vi "GetProbePlanCoordinates.vi"(8 "Use index as X coord":bool=TRUE, 9 "Probe Card Channels":i32=1) -> (0 "file path":string, 2 "OK?":bool, 3 "Array":T1(array[cluster]))   [LabVIEW 2018] (continued)
X=102970.01\ty=15800.93 \nLabel=Strip\t776\tX=103316.84\ty=15902.32 \nLabel=Strip\t777\tX=102964.55\ty=15968.32 \nLabel=Strip\t778\tX=103311.35\ty=16069.84 \nLabel=Strip\t779\tX=102959.04\ty=16135.72 \nLabel=Strip\t780\tX=103305.80\ty=16237.35 \nLabel=Strip\t781\tX=102953.46\ty=16303.11 \nLabel=Strip\t782\tX=103300.19\ty=16404.87 \nLabel=Strip\t783\tX=102947.83\ty=16470.51 \nLabel=Strip\t784\tX=103294.52\ty=16572.38 \nLabel=Strip\t785\tX=102942.14\ty=16637.90 \nLabel=Strip\t786\tX=103288.80\ty=16739.89 \nLabel=Strip\t787\tX=102936.40\ty=16805.30 \nLabel=Strip\t788\tX=103283.02\ty=16907.41 \nLabel=Strip\t789\tX=102930.59\ty=16972.69 \nLabel=Strip\t790\tX=103277.18\ty=17074.92 \nLabel=Strip\t791\tX=102924.73\ty=17140.08 \nLabel=Strip\t792\tX=103271.28\ty=17242.43 \nLabel=Strip\t793\tX=102918.81\ty=17307.47 \nLabel=Strip\t794\tX=103265.33\ty=17409.94 \nLabel=Strip\t795\tX=102912.84\ty=17474.86 \nLabel=Strip\t796\tX=103259.32\ty=17577.45 \nLabel=Strip\t797\tX=102906.80\ty=17642.24 \nLabel=Strip\t798\tX=103253.25\ty=17744.95 \nLabel=Strip\t799\tX=102900.71\ty=17809.63 \nLabel=Strip\t800\tX=103247.12\ty=17912.46 \nLabel=Strip\t801\tX=102894.56\ty=17977.02 \nLabel=Strip\t802\tX=103240.94\ty=18079.96 \nLabel=Strip\t803\tX=102888.35\ty=18144.40 \nLabel=Strip\t804\tX=103234.69\ty=18247.47 \nLabel=Strip\t805\tX=102882.09\ty=18311.78 \nLabel=Strip\t806\tX=103228.39\ty=18414.97 \nLabel=Strip\t807\tX=102875.77\ty=18479.17 \nLabel=Strip\t808\tX=103222.04\ty=18582.47 \nLabel=Strip\t809\tX=102869.39\ty=18646.55 \nLabel=Strip\t810\tX=103215.62\ty=18749.97 \nLabel=Strip\t811\tX=102862.95\ty=18813.93 \nLabel=Strip\t812\tX=103209.15\ty=18917.47 \nLabel=Strip\t813\tX=102856.46\ty=18981.31 \nLabel=Strip\t814\tX=103202.62\ty=19084.97 \nLabel=Strip\t815\tX=102849.90\ty=19148.68 \nLabel=Strip\t816\tX=103196.03\ty=19252.47 \nLabel=Strip\t817\tX=102843.29\ty=19316.06 \nLabel=Strip\t818\tX=103189.38\ty=19419.96 \nLabel=Strip\t819\tX=102836.63\ty=19483.43 \nLabel=Strip\t820\tX=103182.68\ty=19587.46 \nLabel=Strip\t821\tX=102829.90\ty=19650.81 \nLabel=Strip\t822\tX=103175.92\ty=19754.95 \nLabel=Strip\t823\tX=102823.12\ty=19818.18 \nLabel=Strip\t824\tX=103169.10\ty=19922.44 \nLabel=Strip\t825\tX=102816.28\ty=19985.55 \nLabel=Strip\t826\tX=103162.23\ty=20089.93 \nLabel=Strip\t827\tX=102809.38\ty=20152.92 \nLabel=Strip\t828\tX=103155.29\ty=20257.42 \nLabel=Strip\t829\tX=102802.43\ty=20320.29 \nLabel=Strip\t830\tX=103148.30\ty=20424.91 \nLabel=Strip\t831\tX=102795.41\ty=20487.66 \nLabel=Strip\t832\tX=103141.25\ty=20592.39 \nLabel=Strip\t833\tX=102788.34\ty=20655.02 \nLabel=Strip\t834\tX=103134.15\ty=20759.88 \nLabel=Strip\t835\tX=102781.22\ty=20822.39 \nLabel=Strip\t836\tX=103126.98\ty=20927.36 \nLabel=Strip\t837\tX=102774.03\ty=20989.75 \nLabel=Strip\t838\tX=103119.76\ty=21094.85 \nLabel=Strip\t839\tX=102766.79\ty=21157.11 \nLabel=Strip\t840\tX=103112.48\ty=21262.33 \nLabel=Strip\t841\tX=102759.49\ty=21324.47 \nLabel=Strip\t842\tX=103105.14\ty=21429.81 \nLabel=Strip\t843\tX=102752.13\ty=21491.83 \nLabel=Strip\t844\tX=103097.75\ty=21597.28 \nLabel=Strip\t845\tX=102744.71\ty=21659.19 \nLabel=Strip\t846\tX=103090.30\ty=21764.76 \nLabel=Strip\t847\tX=102737.24\ty=21826.54 \nLabel=Strip\t848\tX=103082.79\ty=21932.23 \nLabel=Strip\t849\tX=102729.71\ty=21993.90 \nLabel=Strip\t850\tX=103075.22\ty=22099.71 \nLabel=Strip\t851\tX=102722.12\ty=22161.25 \nLabel=Strip\t852\tX=103067.60\ty=22267.18 \nLabel=Strip\t853\tX=102714.48\ty=22328.60 \nLabel=Strip\t854\tX=103059.91\ty=22434.65 \nLabel=Strip\t855\tX=102706.77\ty=22495.95 \nLabel=Strip\t856\tX=103052.17\ty=22602.12 \nLabel=Strip\t857\tX=102699.01\ty=22663.30 \nLabel=Strip\t858\tX=103044.38\ty=22769.58 \nLabel=Strip\t859\tX=102691.19\ty=22830.64 \nLabel=Strip\t860\tX=103036.52\ty=22937.05 \nLabel=Strip\t861\tX=102683.32\ty=22997.99 \nLabel=Strip\t862\tX=103028.61\ty=23104.51 \nLabel=Strip\t863\tX=102675.38\ty=23165.33 \nLabel=Strip\t864\tX=103020.64\ty=23271.97 \nLabel=Strip\t865\tX=102667.39\ty=23332.67 \nLabel=Strip\t866\tX=103012.61\ty=23439.43 \nLabel=Strip\t867\tX=102659.34\ty=23500.01 \nLabel=Strip\t868\tX=103004.52\ty=23606.89 \nLabel=Strip\t869\tX=102651.24\ty=23667.35 \nLabel=Strip\t870\tX=102996.38\ty=23774.35 \nLabel=Strip\t871\tX=102643.07\ty=23834.68 \nLabel=Strip\t872\tX=102988.18\ty=23941.80 \nLabel=Strip\t873\tX=102634.85\ty=24002.01 \nLabel=Strip\t874\tX=102979.92\ty=24109.26 \nLabel=Strip\t875\tX=102626.57\ty=24169.35 \nLabel=Strip\t876\tX=102971.61\ty=24276.71 \nLabel=Strip\t877\tX=102618.23\ty=24336.68 \nLabel=Strip\t878\tX=102963.23\ty=24444.16 \nLabel=Strip\t879\tX=102609.84\ty=24504.01 \nLabel=Strip\t880\tX=102954.80\ty=24611.60 \nLabel=Strip\t881\tX=102601.39\ty=24671.33 \nLabel=Strip\t882\tX=102946.31\ty=24779.05 \nLabel=Strip\t883\tX=102592.88\ty=24838.66 \nLabel=Strip\t884\tX=102937.76\ty=24946.49 \nLabel=Strip\t885\tX=102584.31\ty=25005.98 \nLabel=Strip\t886\tX=102929.16\ty=25113.93 \nLabel=Strip\t887\tX=102575.68\ty=25173.30 \nLabel=Strip\t888\tX=102920.50\ty=25281.37 \nLabel=Strip\t889\tX=102567.00\ty=25340.62 \nLabel=Strip\t890\tX=102911.78\ty=25448.81 \nLabel=Strip\t891\tX=102558.26\ty=25507.94 \nLabel=Strip\t892\tX=102903.00\ty=25616.25 \nLabel=Strip\t893\tX=102549.47\ty=25675.25 \nLabel=Strip\t894\tX=102894.17\ty=25783.68 \nLabel=Strip\t895\tX=102540.61\ty=25842.56 \nLabel=Strip\t896\tX=102885.28\ty=25951.11 \nLabel=Strip\t897\tX=102531.70\ty=26009.87 \nLabel=Strip\t898\tX=102876.33\ty=26118.54 \nLabel=Strip\t899\tX=102522.73\ty=26177.18 \nLabel=Strip\t900\tX=102867.32\ty=26285.97 \nLabel=Strip\t901\tX=102513.70\ty=26344.49 \nLabel=Strip\t902\tX=102858.25\ty=26453.39 \nLabel=Strip\t903\tX=102504.62\ty=26511.79 \nLabel=Strip\t904\tX=102849.13\ty=26620.82 \nLabel=Strip\t905\tX=102495.47\ty=26679.10 \nLabel=Strip\t906\tX=102839.95\ty=26788.24 \nLabel=Strip\t907\tX=102486.27\ty=26846.40 \nLabel=Strip\t908\tX=102830.71\ty=26955.66 \nLabel=Strip\t909\tX=102477.01\ty=27013.69 \nLabel=Strip\t910\tX=102821.42\ty=27123.08 \nLabel=Strip\t911\tX=102467.70\ty=27180.99 \nLabel=Strip\t912\tX=102812.06\ty=27290.49 \nLabel=Strip\t913\tX=102458.33\ty=27348.28 \nLabel=Strip\t914\tX=102802.65\ty=27457.90 \nLabel=Strip\t915\tX=102448.90\ty=27515.58 \nLabel=Strip\t916\tX=102793.18\ty=27625.31 \nLabel=Strip\t917\tX=102439.41\ty=27682.87 \nLabel=Strip\t918\tX=102783.66\ty=27792.72 \nLabel=Strip\t919\tX=102429.86\ty=27850.15 \nLabel=Strip\t920\tX=102774.07\ty=27960.13 \nLabel=Strip\t921\tX=102420.26\ty=28017.44 \nLabel=Strip\t922\tX=102764.43\ty=28127.53 \nLabel=Strip\t923\tX=102410.60\ty=28184.72 \nLabel=Strip\t924\tX=102754.73\ty=28294.93 \nLabel=Strip\t925\tX=102400.88\ty=28352.00 \nLabel=Strip\t926\tX=102744.98\ty=28462.33 \nLabel=Strip\t927\tX=102391.10\ty=28519.28 \nLabel=Strip\t928\tX=102735.16\ty=28629.73 \nLabel=Strip\t929\tX=102381.27\ty=28686.56 \nLabel=Strip\t930\tX=102725.29\ty=28797.12 \nLabel=Strip\t931\tX=102371.38\ty=28853.83 \nLabel=Strip\t932\tX=102715.36\ty=28964.51 \nLabel=Strip\t933\tX=102361.43\ty=29021.10 \nLabel=Strip\t934\tX=102705.38\ty=29131.90 \nLabel=Strip\t935\tX=102351.42\ty=29188.37 \nLabel=Strip\t936\tX=102695.33\ty=29299.29 \nLabel=Strip\t937\tX=102341.36\ty=29355.63 \nLabel=Strip\t938\tX=102685.23\ty=29466.68 \nLabel=Strip\t939\tX=102331.24\ty=29522.90 \nLabel=Strip\t940\tX=102675.07\ty=29634.06 \nLabel=Strip\t941\tX=102321.06\ty=29690.16 \nLabel=Strip\t942\tX=102664.85\ty=29801.44 \nLabel=Strip\t943\tX=102310.82\ty=29857.42 \nLabel=Strip\t944\tX=102654.58\ty=29968.82 \nLabel=Strip\t945\tX=102300.53\ty=30024.67 \nLabel=Strip\t946\tX=102644.24\ty=30136.19 \nLabel=Strip\t947\tX=102290.17\ty=30191.93 \nLabel=Strip\t948\tX=102633.85\ty=30303.56 \nLabel=Strip\t949\tX=102279.77\ty=30359.18 \nLabel=Strip\t950\tX=102623.41\ty=30470.93 \nLabel=Strip\t951\tX=102269.30\ty=30526.43 \nLabel=Strip\t952\tX=102612.90\ty=30638.30 \nLabel=Strip\t953\tX=102258.77\ty=30693.67 \nLabel=Strip\t954\tX=102602.34\ty=30805.66 \nLabel=Strip\t955\tX=102248.19\ty=30860.92 \nLabel=Strip\t956\tX=102591.72\ty=30973.03 \nLabel=Strip\t957\tX=102237.55\ty=31028.16 \nLabel=Strip\t958\tX=102581.04\ty=31140.39 \nLabel=Strip\t959\tX=102226.85\ty=31195.40 \nLabel=Strip\t960\tX=102570.30\ty=31307.74 \nLabel=Strip\t961\tX=102216.10\ty=31362.63 \nLabel=Strip\t962\tX=102559.51\ty=31475.10 \nLabel=Strip\t963\tX=102205.29\ty=31529.87 \nLabel=Strip\t964\tX=102548.66\ty=31642.45 \nLabel=Strip\t965\tX=102194.42\ty=31697.10 \nLabel=Strip\t966\tX=102537.75\ty=31809.80 \nLabel=Strip\t967\tX=102183.49\ty=31864.32 \nLabel=Strip\t968\tX=102526.78\ty=31977.14 \nLabel=Strip\t969\tX=102172.51\ty=32031.55 \nLabel=Strip\t970\tX=102515.76\ty=32144.49 \nLabel=Strip\t971\tX=102161.46\ty=32198.77 \nLabel=Strip\t972\tX=102504.68\ty=32311.83 \nLabel=Strip\t973\tX=102150.36\ty=32365.99 \nLabel=Strip\t974\tX=102493.54\ty=32479.16 \nLabel=Strip\t975\tX=102139.20\ty=32533.21 \nLabel=Strip\t976\tX=102482.34\ty=32646.50 \nLabel=Strip\t977\tX=102127.99\ty=32700.42 \nLabel=Strip\t978\tX=102471.09\ty=32813.83 \nLabel=Strip\t979\tX=102116.72\ty=32867.63 \nLabel=Strip\t980\tX=102459.78\ty=32981.16 \nLabel=Strip\t981\tX=102105.39\ty=33034.84 \nLabel=Strip\t982\tX=102448.41\ty=33148.49 \nLabel=Strip\t983\tX=102094.00\ty=33202.04 \nLabel=Strip\t984\tX=102436.98\ty=33315.81 \nLabel=Strip\t985\tX=102082.55\ty=33369.25 \nLabel=Strip\t986\tX=102425.50\ty=33483.13 \nLabel=Strip\t987\tX=102071.05\ty=33536.44 \nLabel=Strip\t988\tX=102413.95\ty=33650.45 \nLabel=Strip\t989\tX=102059.49\ty=33703.64 \nLabel=Strip\t990\tX=102402.35\ty=33817.76 \nLabel=Strip\t991\tX=102047.87\ty=33870.83 \nLabel=Strip\t992\tX=102390.70\ty=33985.07 \nLabel=Strip\t993\tX=102036.20\ty=34038.02 \nLabel=Strip\t994\tX=102378.98\ty=34152.38 \nLabel=Strip\t995\tX=102024.46\ty=34205.21 \nLabel=Strip\t996\tX=102367.21\ty=34319.69 \nLabel=Strip\t997\tX=102012.67\ty=34372.40 \nLabel=Strip\t998\tX=102355.38\ty=34486.99 \nLabel=Strip\t999\tX=102000.82\ty=34539.58 \nLabel=Strip\t1000\tX=102343.49\ty=34654.29 \nLabel=Strip\t1001\tX=101988.92\ty=34706.76 \nLabel=Strip\t1002\tX=102331.54\ty=34821.59 \nLabel=Strip\t1003\tX=101976.95\ty=34873.93 \nLabel=Strip\t1004\tX=102319.54\ty=34988.88 \nLabel=Strip\t1005\tX=101964.93\ty=35041.10 \nLabel=Strip\t1006\tX=102307.48\ty=35156.17 \nLabel=Strip\t1007\tX=101952.85\ty=35208.27 \nLabel=Strip\t1008\tX=102295.36\ty=35323.46 \nLabel=Strip\t1009\tX=101940.72\ty=35375.44 \nLabel=Strip\t1010\tX=102283.19\ty=35490.74 \nLabel=Strip\t1011\tX=101928.52\ty=35542.60 \nLabel=Strip\t1012\tX=102270.95\ty=35658.02 \nLabel=Strip\t1013\tX=101916.27\ty=35709.76 \nLabel=Strip\t1014\tX=102258.66\ty=35825.30 \nLabel=Strip\t1015\tX=101903.96\ty=35876.92 \nLabel=Strip\t1016\tX=102246.31\ty=35992.57 \nLabel=Strip\t1017\tX=101891.59\ty=36044.07 \nLabel=Strip\t1018\tX=102233.91\ty=36159.84 \nLabel=Strip\t1019\tX=101879.17\ty=36211.22 \nLabel=Strip\t1020\tX=102221.44\ty=36327.11 \nLabel=Strip\t1021\tX=101866.69\ty=36378.37 \nLabel=Strip\t1022\tX=102208.92\ty=36494.38 \nLabel=Strip\t1023\tX=101854.15\ty=36545.51 \nLabel=Strip\t1024\tX=102196.34\ty=36661.64 \nLabel=Strip\t1025\tX=101841.55\ty=36712.65 \nLabel=Strip\t1026\tX=102183.70\ty=36828.90 \nLabel=Strip\t1027\tX=101828.90\ty=36879.79 \nLabel=Strip\t1028\tX=102171.00\ty=36996.22 \nLabel=Strip\t1029\tX=101816.19\ty=37046.92 \nLabel=Strip\t1030\tX=102158.26\ty=37163.40 \nLabel=Strip\t1031\tX=101803.42\ty=37214.05 \nLabel=Strip\t1032\tX=102145.45\ty=37330.65 \nLabel=Strip\t1033\tX=101790.59\ty=37381.18 \nLabel=Strip\t1034\tX=102132.58\ty=37497.89 \nLabel=Strip\t1035\tX=101777.71\ty=37548.30 \nLabel=Strip\t1036\tX=102119.66\ty=37665.14 \nLabel=Strip\t1037\tX=101764.76\ty=37715.42 \nLabel=Strip\t1038\tX=102106.67\ty=37832.37 \nLabel=Strip\t1039\tX=101751.76\ty=37882.54 \nLabel=Strip\t1040\tX=102093.63\ty=37999.61 \nLabel=Strip\t1041\tX=101738.71\ty=38049.65 \nLabel=Strip\t1042\tX=102080.54\ty=38166.84 \nLabel=Strip\t1043\tX=101725.59\ty=38216.76 \nLabel=Strip\t1044\tX=102067.38\ty=38334.07 \nLabel=Strip\t1045\tX=101712.42\ty=38383.86 \nLabel=Strip\t1046\tX=102054.17\ty=38501.29 \nLabel=Strip\t1047\tX=101699.19\ty=38550.97 \nLabel=Strip\t1048\tX=102040.90\ty=38668.51 \nLabel=Strip\t1049\tX=101685.90\ty=38718.07 \nLabel=Strip\t1050\tX=102027.57\ty=38835.73 \nLabel=Strip\t1051\tX=101672.56\ty=38885.16 \nLabel=Strip\t1052\tX=102014.19\ty=39002.94 \nLabel=Strip\t1053\tX=101659.16\ty=39052.25 \nLabel=Strip\t1054\tX=102000.74\ty=39170.15 \nLabel=Strip\t1055\tX=101645.69\ty=39219.34 \nLabel=Strip\t1056\tX=101987.24\ty=39337.36 \nLabel=Strip\t1057\tX=101632.18\ty=39386.43 \nLabel=Strip\t1058\tX=101973.68\ty=39504.56 \nLabel=Strip\t1059\tX=101618.60\ty=39553.51 \nLabel=Strip\t1060\tX=101960.07\ty=39671.76 \nLabel=Strip\t1061\tX=101604.97\ty=39720.58 \nLabel=Strip\t1062\tX=101946.39\ty=39838.95 \nLabel=Strip\t1063\tX=101591.28\ty=39887.66 \nLabel=Strip\t1064\tX=101932.66\ty=40006.14 \nLabel=Strip\t1065\tX=101577.53\ty=40054.73 \nLabel=Strip\t1066\tX=101918.87\ty=40173.33 \nLabel=Strip\t1067\tX=101563.73\ty=40221.79 \nLabel=Strip\t1068\tX=101905.03\ty=40340.52 \nLabel=Strip\t1069\tX=101549.86\ty=40388.86 \nLabel=Strip\t1070\tX=101891.12\ty=40507.70 \nLabel=Strip\t1071\tX=101535.94\ty=40555.92 \nLabel=Strip\t1072\tX=101877.16\ty=40674.87 \nLabel=Strip\t1073\tX=101521.96\ty=40722.97 \nLabel=Strip\t1074\tX=101863.14\ty=40842.05 \nLabel=Strip\t1075\tX=101507.93\ty=40890.02 \nLabel=Strip\t1076\tX=101849.07\ty=41009.21 \nLabel=Strip\t1077\tX=101493.83\ty=41057.07 \nLabel=Strip\t1078\tX=101834.93\ty=41176.38 \nLabel=Strip\t1079\tX=101479.68\ty=41224.11 \nLabel=Strip\t1080\tX=101820.74\ty=41343.54 \nLabel=Strip\t1081\tX=101465.48\ty=41391.15 \nLabel=Strip\t1082\tX=101806.49\ty=41510.70 \nLabel=Strip\t1083\tX=101451.21\ty=41558.19 \nLabel=Strip\t1084\tX=101792.18\ty=41677.85 \nLabel=Strip\t1085\tX=101436.89\ty=41725.22 \nLabel=Strip\t1086\tX=101777.82\ty=41845.00 \nLabel=Strip\t1087\tX=101422.51\ty=41892.25 \nLabel=Strip\t1088\tX=101763.40\ty=42012.15 \nLabel=Strip\t1089\tX=101408.07\ty=42059.27 \nLabel=Strip\t1090\tX=101748.92\ty=42179.29 \nLabel=Strip\t1091\tX=101393.57\ty=42226.29 \nLabel=Strip\t1092\tX=101734.38\ty=42346.43 \nLabel=Strip\t1093\tX=101379.02\ty=42393.31 \nLabel=Strip\t1094\tX=101719.79\ty=42513.56 \nLabel=Strip\t1095\tX=101364.41\ty=42560.32 \nLabel=Strip\t1096\tX=101705.13\ty=42680.69 \nLabel=Strip\t1097\tX=101349.74\ty=42727.33 \nLabel=Strip\t1098\tX=101690.42\ty=42847.81 \nLabel=Strip\t1099\tX=101335.01\ty=42894.33 \nLabel=Strip\t1100\tX=101675.66\ty=43014.94 \nLabel=Strip\t1101\tX=101320.23\ty=43061.33 \nLabel=Strip\t1102\tX=101660.83\ty=43182.05 \nLabel=Strip\t1103\tX=101305.39\ty=43228.33 \nLabel=Strip\t1104\tX=101645.95\ty=43349.17 \nLabel=Strip\t1105\tX=101290.49\ty=43395.32 \nLabel=Strip\t1106\tX=101631.01\ty=43516.28 \nLabel=Strip\t1107\tX=101275.53\ty=43562.31 \nLabel=Strip\t1108\tX=101616.01\ty=43683.38 \nLabel=Strip\t1109\tX=101260.52\ty=43729.29 \nLabel=Strip\t1110\tX=101600.96\ty=43850.48 \nLabel=Strip\t1111\tX=101245.45\ty=43896.27 \nLabel=Strip\t1112\tX=101585.84\ty=44017.58 \nLabel=Strip\t1113\tX=101230.32\ty=44063.25 \nLabel=Strip\t1114\tX=101570.67\ty=44184.67 \nLabel=Strip\t1115\tX=101215.13\ty=44230.22 \nLabel=Strip\t1116\tX=101555.44\ty=44351.76 \nLabel=Strip\t1117\tX=101199.89\ty=44397.19 \nLabel=Strip\t1118\tX=101540.15\ty=44518.94 \nLabel=Strip\t1119\tX=101184.59\ty=44564.15 \nLabel=Strip\t1120\tX=101524.81\ty=44685.93 \nLabel=Strip\t1121\tX=101169.23\ty=44731.11 \nLabel=Strip\t1122\tX=101509.41\ty=44853.00 \nLabel=Strip\t1123\tX=101153.81\ty=44898.06 \nLabel=Strip\t1124\tX=101493.96\ty=45020.07 \nLabel=Strip\t1125\tX=101138.34\ty=45065.01 \nLabel=Strip\t1126\tX=101478.44\ty=45187.14 \nLabel=Strip\t1127\tX=101122.81\ty=45231.96 \nLabel=Strip\t1128\tX=101462.87\ty=45354.20 \nLabel=Strip\t1129\tX=101107.22\ty=45398.90 \nLabel=Strip\t1130\tX=101447.23\ty=45521.26 \nLabel=Strip\t1131\tX=101091.57\ty=45565.83 \nLabel=Strip\t1132\tX=101431.55\ty=45688.32 \nLabel=Strip\t1133\tX=101075.87\ty=45732.77 \nLabel=Strip\t1134\tX=101415.80\ty=45855.37 \nLabel=Strip\t1135\tX=101060.11\ty=45899.70 \nLabel=Strip\t1136\tX=101400.00\ty=46022.41 \nLabel=Strip\t1137\tX=101044.29\ty=46066.62 \nLabel=Strip\t1138\tX=101384.13\ty=46189.45 \nLabel=Strip\t1139\tX=101028.41\ty=46233.54 \nLabel=Strip\t1140\tX=101368.22\ty=46356.49 \nLabel=Strip\t1141\tX=101012.48\ty=46400.45 \nLabel=Strip\t1142\tX=101352.24\ty=46523.52 \nLabel=Strip\t1143\tX=100996.48\ty=46567.36 \nLabel=Strip\t1144\tX=101336.20\ty=46690.55 \nLabel=Strip\t1145\tX=100980.43\ty=46734.27 \nLabel=Strip\t1146\tX=101320.11\ty=46857.57 \nLabel=Strip\t1147\tX=100964.33\ty=46901.17 \nLabel=Strip\t1148\tX=101303.96\ty=47024.59 \nLabel=Strip\t1149\tX=100948.16\ty=47068.07 \nLabel=Strip\t1150\tX=101287.76\ty=47191.60 \nLabel=Strip\t1151\tX=100931.94\ty=47234.96 \nLabel=Strip\t1152\tX=101271.49\ty=47358.61 \nLabel=Strip\t1153\tX=100915.66\ty=47401.85 \nLabel=Strip\t1154\tX=101255.17\ty=47525.62 \n"
  in  "Stop Button":bool
  in  "OK Button":bool
  in  "Region":u16(ring)=3
  out "Coordinates":string[][](table)
  # "ProbePlan Coordinates"
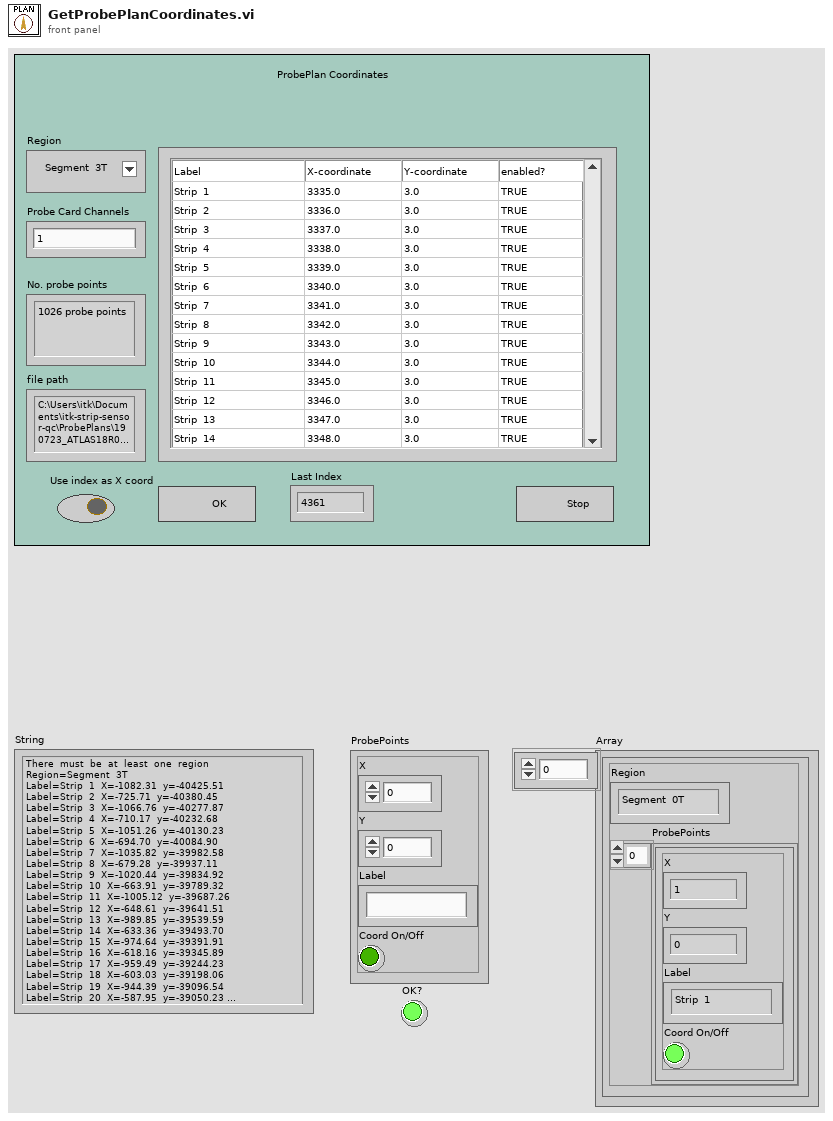
[diagram p1: front panel]
types:
  T1 = cluster{"Region":string, "ProbePoints":cluster{"X":dbl, "Y":dbl, "Label":string, "Coord On/Off":bool}[]}[]
  T2 = cluster{"X":dbl, "Y":dbl, "Label":string, "Coord On/Off":bool}
  T3 = cluster{"Region":string, "ProbePoints":cluster{"X":dbl, "Y":dbl, "Label":string, bool}[]}[]
  T4 = enum16{"open", "replace", "create", "open or create", "replace or create", "replace or create with confirmation"}
  T5 = cluster{"X":dbl, "Y":dbl, "Label":string, bool}[]
  T6 = cluster{"Bias Supply":refnum<class "SupplyControl.lvclass">, "SMU":refnum<class "SupplyControl.lvclass">, "LCR":refnum<class "LCRControl.lvclass">, "Probe Card Channels":i32, "Bias Voltage [V]":dbl, "First strip":i32, "Last strip":i32, "Base Voltage [V]":dbl, "Base Ramp Step [V]":dbl, "Base Ramp Interval [ms]":u32, "High Voltage [V]":dbl, "High Ramp Step [V]":dbl, "High Ramp Interval [ms]":u32, "Single Needle":bool, "Temperature Readout":enum16{"Read Arduino", "Enter manually"}, "Arduino":refnum<class "ArduinoControl.lvclass">, "Fraction of good strips [%]":dbl, "ProbeStation":refnum<class "ProbeStationControl.lvclass">, "AC frequency [Hz]":i32, "Switching":refnum<class "Switching.lvclass">, "Matrix used?":bool, "Matrix X Channels":cluster{"Bias Supply / SMU LO":i32, "Bias Supply / SMU HI":i32, "CV Box LO":i32, "CV Box HI":i32, "CV Box LO IN":i32, "CV Box HI IN":i32, "Volt meter LO":i32, "Volt meter HI":i32, "Mux1 C1":i32, "Mux1 C2":i32, "Mux2 C1":i32, "Mux2 C2":i32}, "Pinholes Y/N":bool, "Capacitance Y/N":bool, "Resistance Y/N":bool}
  T7 = cluster{"submatch 1":string, "ProbePoints":cluster{"X":dbl, "Y":dbl, "Label":string, bool}[]}
  T8 = cluster{"submatch 1":string, "ProbePoints":cluster{"X":dbl, "Y":dbl, "Label":string, bool}[]}[]
  T9 = cluster{"Region":string, "ProbePoints":cluster{"X":dbl, "Y":dbl, "Label":string, bool}[]}
  T10 = cluster{"X":dbl, "Y":dbl, "Label":string, "Coord On/Off":bool}[]
  T11 = cluster{"Region":string, cluster{"X":dbl, "Y":dbl, "Label":string, "Coord On/Off":bool}[]}
  T12 = cluster{"Strip Number OUT":i32, "X0":i32, "Y0":i32, "X1":i32, "Y1":i32, "Xref":dbl, "Yref":dbl, "ProbePlan type":u32, "Inner pads offset":ext, "Outer pads offset":ext, "l_inner":ext, "l_outer":ext, "strip numbering":u16, "Device Orientation":ext, "Stagger offset":i32, "Yoffset":dbl, "Strip pitch":dbl, "Fiducail separation":dbl, "Radius":ext, "Relative strip angles":dbl, "Probeplan description":string, "ProbePlan array":cluster{"Region":string, "ProbePoints":cluster{"X":dbl, "Y":dbl, "Label":string, "CardViable?":bool}[]}[], "Test ProbePoints":cluster{"Regions Enabled":bool[], "From index":u32[], "To index":u32[]}}
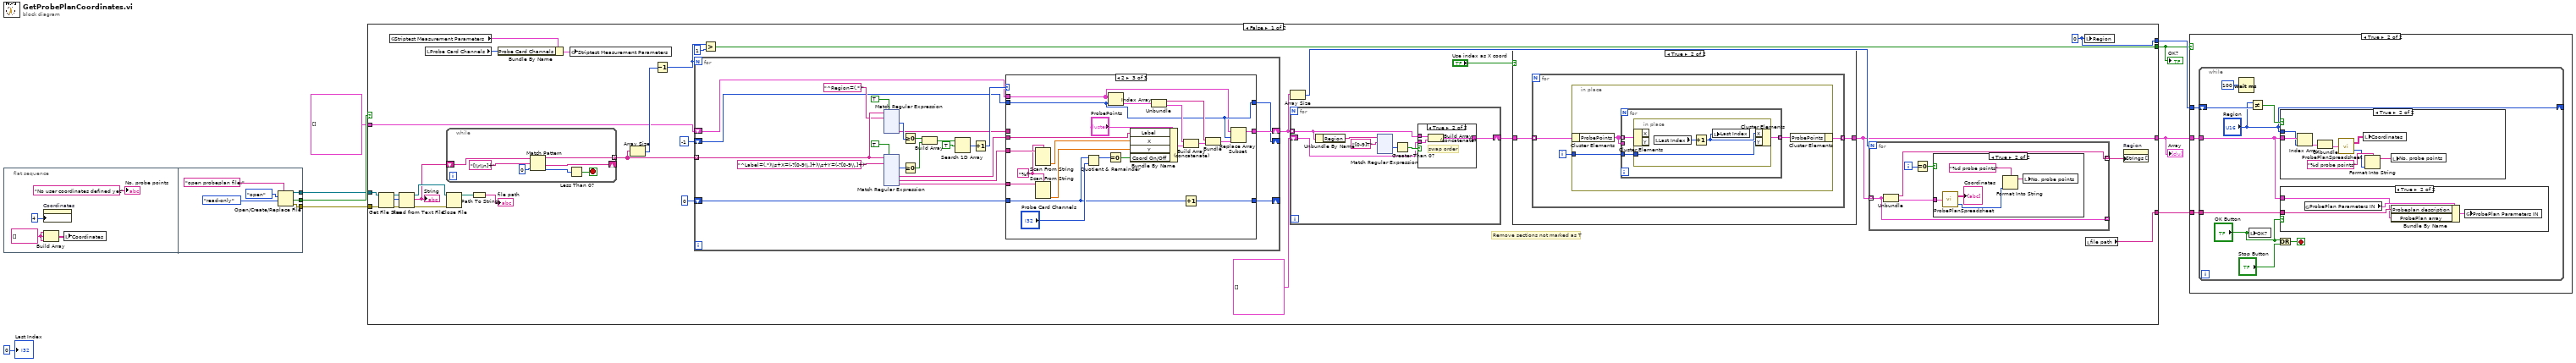
[diagram p0: block diagram]
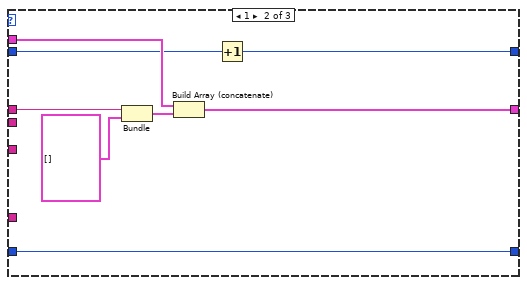
[diagram p9: hidden frame]
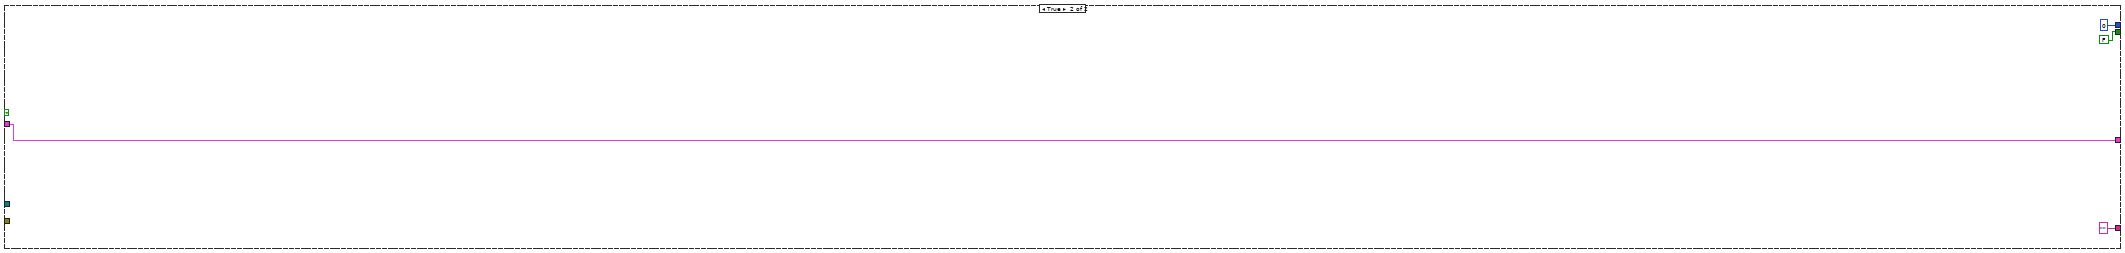
[diagram p10: hidden frame]
diagram:
  n1 = flat-sequence {
    tunnel: [w16] -> w9
    tunnel: [w15] -> w7
    tunnel: [w14] -> w8
    frame #0 {
      w13 = string[] []
      n2 = property on="Coordinates" class="Tbl (strict)"("Number of Columns"=4) -> ()  [unwired: 2 in, 2 out]
      n3 = Build Array(w13, w13, w13) -> (w12:string[][])
      n4 = local write "Coordinates"(w12) -> ()
      "No. probe points" <- "No user coordinates defined yet" ("String 2")
    }
    frame #1 {
      n5 = Open/Create/Replace File(prompt="open probeplan file:", operation (0:open)=T4."open", access (0:read/write)=enum16{"read/write", "read-only", "write-only"}."read-only") -> (refnum out=w14:refnum<file>, cancelled=w16:bool, error out=w15:errorcluster)  [unwired: 3 in]
    }
  }
  n6 = case shown="False" w9 {
    tunnel: T3 [] ("Array") -> [w36 w499]
    tunnel: w8 -> [w49 _]
    tunnel: w7 -> [w44 _]
    tunnel: [w21 w499] -> w5
    tunnel: [w34 0] -> w4
    tunnel: [w30 FALSE] -> w3
    tunnel: [w29 ""] -> w6
    frame False {
      w34 = 0
      # "Remove sections not marked as T"
      n7 = Get File Size(file=w49, error in=w44) -> (refnum out=w48:refnum<file>, size (in bytes)=w43:i64, 0:w46:errorcluster)
      n8 = global read "QC_MeasurementSetup.vi" "Striptest Measurement Parameters"() -> (w26:T6)
      n9 = Read from Text File(file (use dialog)=w48, count=w43, error in=w46) -> (refnum out=w47:refnum<file>, text=w40:string, error out=w45:errorcluster)  [unwired: 1 in, 1 out]
      "String" <- w40
      n10 = local read "Probe Card Channels"() -> (w27:i32)
      n11 = while {
        shift-right: [w492] -> _
        shift-left: w40 -> [w495]
        tunnel: [w489] -> w38 mode=indexing
        stop <- w491 stop-if-true
        n12 = Match Pattern(string=w495, regular expression="[\\r\\n]+", offset (0)=0) -> (before substring=w489:string, after substring=w492:string, offset past match=w490:i32)  [unwired: 1 out]
        n13 = Less Than 0?(x=w490) -> (x < 0?=w491:bool)
      }
      n14 = Close File(refnum=w47, error in=w45) -> (path=w42:path)  [unwired: 1 out]
      n15 = Path To String(path=w42) -> (string=→"file path":string)
      n16 = Bundle By Name(cluster=w26, "Probe Card Channels"=w27) -> (w25:T6)
      n17 = global write "QC_MeasurementSetup.vi" "Striptest Measurement Parameters"(w25) -> ()
      n18 = Array Size(array=w38) -> (size(s)=w39:i32)
      n19 = Decrement(x=w39) -> (x-1=w31:i32)
      n20 = for {
        N: w31 -> [_]
        tunnel: w38 -> [w216] mode=indexing
        shift-right: [w202] -> _
        shift-left: -1 -> [w203]
        shift-right: [w204] -> w24
        shift-left: w36 -> [w205]
        shift-right: [w201] -> _
        shift-left: 0 -> [w200]
        n21 = xnode "Match Regular Expression"("input string"=w216, "regular expression"="^Region=(.*)", "ignore case? (F)"=TRUE) -> ("offset past match"=w213:i32, "submatch 1"=w206:string)  [unwired: 3 in, 4 out]
        n22 = xnode "Match Regular Expression"("input string"=w216, "regular expression"="^Label=(.*)\\s+X=(-?[0-9\\.]+)\\s+Y=(-?[0-9\\.]+)", "ignore case? (F)"=TRUE) -> ("offset past match"=w219:i32, "submatch 1"=w220:string, "submatch 2"=w217:string, "submatch 3"=w218:string)  [unwired: 3 in, 4 out]
        n23 = Greater Or Equal To 0?(x=w213) -> (x >= 0?=w212:bool)
        n24 = Greater Or Equal To 0?(x=w219) -> (x >= 0?=w211:bool)
        n25 = Build Array(w212, w211) -> (w210:bool[])
        n26 = Search 1D Array(1D array=w210, element=TRUE) -> (index of element=w208:i32)  [unwired: 1 in]
        n27 = Increment(x=w208) -> (x+1=w207:i32)
        n28 = case shown="2" w207 {
          tunnel: w220 -> [_ _ w367]
          tunnel: w218 -> [_ _ w365]
          tunnel: w217 -> [_ _ w366]
          tunnel: w206 -> [_ w349 _]
          tunnel: w205 -> [w341 w347 w361]
          tunnel: [w341 w345 w359] -> w204
          tunnel: w203 -> [w340 w344 w362]
          tunnel: [w340 w343 w362] -> w202
          tunnel: [w339 w342 w353] -> w201
          tunnel: w200 -> [w339 w342 w352]
          frame 0, Default {
          }
          frame 1 {
            n29 = Bundle("submatch 1"=w349, "ProbePoints"=T5 []) -> (w346:T7)  [unwired: 1 in]
            n30 = Build Array (concatenate)(w347, w346) -> (w345:T8)
            n31 = Increment(x=w344) -> (x+1=w343:i32)
          }
          frame 2 {
            w364 = "%f" ("format string")
            n32 = Scan From String(format string=w364, input string=w366) -> (output 1=w350:dbl)  [unwired: 3 in, 3 out]
            n33 = Scan From String(format string=w364, input string=w365) -> (output 1=w351:dbl)  [unwired: 3 in, 3 out]
            n34 = Quotient & Remainder(x=w352, y="Probe Card Channels") -> (x-y*floor(x/y)=w356:i32)  [unwired: 1 out]
            n35 = Equal To 0?(x=w356) -> (x = 0?=w354:bool)
            n36 = Index Array(array=w361, index=w362) -> (element=w370:T9)
            n37 = Bundle By Name(cluster="ProbePoints", "Label"=w367, "X"=w350, "Y"=w351, "Coord On/Off"=w354) -> (w357:T2)
            n38 = Unbundle(w370) -> ("Region"=w369:string, "ProbePoints"=w368:T5)
            n39 = Increment(x=w352) -> (x+1=w353:i32)
            n40 = Build Array (concatenate)(w368, w357) -> (w363:T10)
            n41 = Bundle("Region"=w369, w363) -> (w360:T11)  [unwired: 1 in]
            n42 = Replace Array Subset(array=w361, new element=w360, index=w362) -> (w359:T3)
          }
        }
      }
      n43 = Greater?(x=w31, y=1) -> (0:w30:bool)
      n44 = Array Size(array=w24) -> (size(s)=w35:i32)
      n45 = for {
        tunnel: w24 -> [w67] mode=indexing
        shift-right: [w65] -> w22
        shift-left: T3 [] ("Array") -> [w66]
        n46 = Unbundle By Name(w67) -> ("Region"=w70:string)
        n47 = xnode "Match Regular Expression"("input string"=w70, "regular expression"="[0-9]T") -> ("offset past match"=w69:i32)  [unwired: 4 in, 4 out]
        n48 = Greater Than 0?(x=w69) -> (x > 0?=w68:bool)
        n49 = case shown="True" w68 {
          tunnel: w67 -> [_ w74]
          tunnel: w66 -> [w72 w75]
          tunnel: [w72 w73] -> w65
          frame False {
            # "throw\naway"
          }
          frame True {
            # "swap order"
            n50 = Build Array (concatenate)(w74, w75) -> (w73:T3)
          }
        }
      }
      n51 = case shown="True" "Use index as X coord" {
        tunnel: w22 -> [w50 w52]
        tunnel: [w50 w51] -> w21
        frame False {
        }
        frame True {
          n52 = for {
            tunnel: w52 -> [w55] mode=indexing
            tunnel: [w54] -> w51 mode=indexing
            i -> [w53]
            n53 = in-place {
              in-place-border: w53 -> [w56]
              n54 = in-place-cluster #1(w55) -> ("ProbePoints"=w57:T5)
              n55 = for {
                tunnel: w57 -> [w61] mode=indexing
                tunnel: [w60] -> w58 mode=indexing
                tunnel: w57 -> [_]
                tunnel: w56 -> [w59]
                n56 = in-place {
                  in-place-border: w59 -> [w63]
                  n57 = in-place-cluster #2(w61) -> ()  [unwired: 2 out]
                  n58 = local read "Last Index"() -> (w64:i32)
                  n59 = Increment(x=w64) -> (x+1=w62:i32)
                  n60 = local write "Last Index"(w62) -> ()
                  n61 = in-place-cluster #2("X"=w62, "Y"=w63) -> (w60:cluster{"X":dbl, "Y":dbl, "Label":string, bool})
                }
              }
              n62 = in-place-cluster #1("ProbePoints"=w58) -> (w54:T9)
            }
          }
        }
      }
      n63 = for {
        N: w35 -> [_]
        tunnel: [w190] -> _ mode=indexing
        tunnel: [w194] -> w33 mode=indexing
        tunnel: w21 -> [w190] mode=indexing
        i -> [w192]
        n64 = Unbundle(w190) -> ("Region"=w194:string, "ProbePoints"=w193:T5)
        n65 = Equal To 0?(x=w192) -> (x = 0?=w191:bool)
        n66 = case shown="True" w191 {
          tunnel: w193 -> [_ w197]
          frame False {
          }
          frame True {
            n67 = call "ProbePlanSpreadsheet.vi"("ProbePoints"=w197) -> ("Coordinates"=→"Coordinates":string[][], "Number of ProbePoints"=w196:i32)
            n68 = Format Into String(format string="%d probe points", w196) -> (resulting string=w198:string)  [unwired: 2 in, 1 out]
            n69 = local write "No. probe points"(w198) -> ()
          }
        }
      }
      n70 = local write "Region"(w34) -> ()
      n71 = local read "file path"() -> (w29:string)
      n72 = property on="Region" class="Ring (strict)"("Strings []"=w33) -> ()  [unwired: 2 in, 2 out]
    }
    frame True {
    }
  }
  "Array" <- w5
  "OK?" <- w3
  n73 = case shown="True" w3 {
    tunnel: w4 -> [_ w502]
    tunnel: w5 -> [_ w501]
    tunnel: w6 -> [_ w500]
    frame False {
    }
    frame True {
      n74 = while {
        shift-right: ["Region"] -> _
        shift-left: w502 -> [w510]
        tunnel: w501 -> [w507]
        tunnel: w500 -> [w506]
        stop <- w511 stop-if-true
        n75 = Wait (ms)(milliseconds to wait=u32 100) -> ()  [unwired: 1 out]
        n76 = local write "OK?"("OK Button") -> ()
        n77 = Not Equal?(x="Region", y=w510) -> (x != y?=w509:bool)
        n78 = Or(x="OK Button", y="Stop Button") -> (x .or. y?=w511:bool)
        n79 = case shown="True" w509 {
          tunnel: w507 -> [_ w523]
          tunnel: "Region" -> [_ w521]
          frame False {
          }
          frame True {
            n80 = Index Array(array=w523, index=w521) -> (element=w522:T9)
            n81 = Unbundle(w522) -> ("ProbePoints"=w518:T5)  [unwired: 1 out]
            n82 = call "ProbePlanSpreadsheet.vi"("ProbePoints"=w518) -> ("Coordinates"=w516:string[][], "Number of ProbePoints"=w517:i32)
            n83 = local write "Coordinates"(w516) -> ()
            n84 = Format Into String(format string="%d probe points", w517) -> (resulting string=w520:string)  [unwired: 2 in, 1 out]
            n85 = local write "No. probe points"(w520) -> ()
          }
        }
        n86 = case shown="True" "OK Button" {
          tunnel: w507 -> [_ w512]
          tunnel: w506 -> [_ w513]
          frame False {
          }
          frame True {
            n87 = global read "ProbePlanParams.vi" "ProbePlan Parameters IN"() -> (w515:T12)
            n88 = Bundle By Name(cluster=w515, "Probeplan description"=w513, "ProbePlan array"=w512) -> (w514:T12)
            n89 = global write "ProbePlanParams.vi" "ProbePlan Parameters IN"(w514) -> ()
          }
        }
      }
    }
  }
  "Last Index" <- 0 ("Index")
